vi "SSC Digital Frequency Counter Configure Measurement Time.vi"(0 "Digital SSC in":T1[](array[typedef]), 5 "Measurement Time (s)":dbl, 11 "error in":errorcluster) -> (4 "Digital SSC out":T1[](array[typedef]), 15 "error out":errorcluster)   [LabVIEW 2020]
doc: "Configures the measurement time for the frequency counter on the specified pin(s) and pin group(s)."
uses:
  SSC Digital.ctl
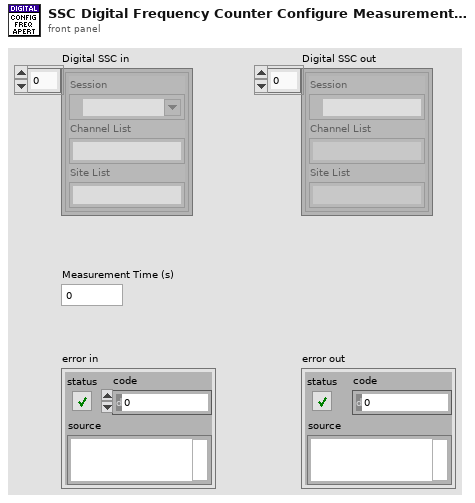
[diagram p1: front panel]
types:
  T1 = typedef "SSC Digital.ctl" = cluster{"Session":refnum<k15>, "Channel List":string, "Site List":string}
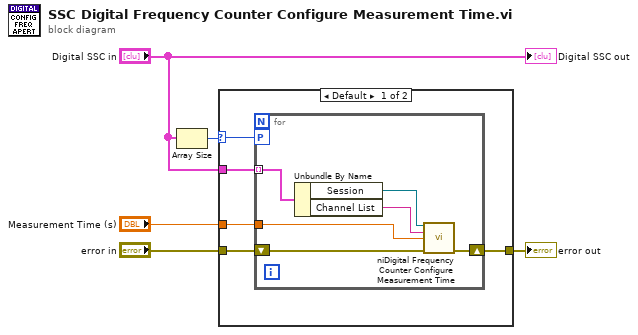
[diagram p0: block diagram]
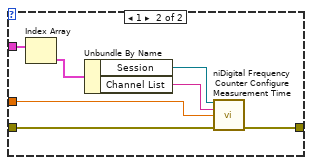
[diagram p2: hidden frame]
diagram:
  n1 = Array Size(array="Digital SSC in") -> (size(s)=w2:i32)
  n2 = case shown="Default" w2 {
    selector: w2 -> [w7 _]
    tunnel: "error in" -> [w10 w23]
    tunnel: "Measurement Time (s)" -> [w9 w22]
    tunnel: [w8 w21] -> w3
    tunnel: "Digital SSC in" -> [w6 w20]
    frame Default {
      n3 = for {
        workers-P: w7 -> [_]
        tunnel: w6 -> [w13] mode=indexing
        tunnel: w9 -> [w11]
        shift-right: [w15] -> w8
        shift-left: w10 -> [w16]
        n4 = Unbundle By Name(w13) -> ("Session"=w14:refnum<k15>, "Channel List"=w12:string)
        n5 = call <instrlib>:"niDigital Frequency Counter Configure Measurement Time.vi"("instrument handle"=w14, "channel list"=w12, "measurement time (s)"=w11, "error in"=w16) -> ("error out"=w15:errorcluster)  [unwired: 10 in, 1 out]
      }
    }
    frame 1 {
      n6 = Index Array(array=w20) -> (element=w17:T1)  [unwired: 1 in]
      n7 = Unbundle By Name(w17) -> ("Session"=w19:refnum<k15>, "Channel List"=w18:string)
      n8 = call <instrlib>:"niDigital Frequency Counter Configure Measurement Time.vi"("instrument handle"=w19, "channel list"=w18, "measurement time (s)"=w22, "error in"=w23) -> ("error out"=w21:errorcluster)  [unwired: 10 in, 1 out]
    }
  }
  "error out" <- w3
  "Digital SSC out" <- "Digital SSC in"
